vi "Circumference of Circle.vi"() -> ()   [LabVIEW 2020]
panel:
  out "Circumference":dbl
  in  "Radius":dbl
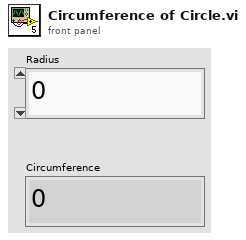
[diagram p1: front panel]
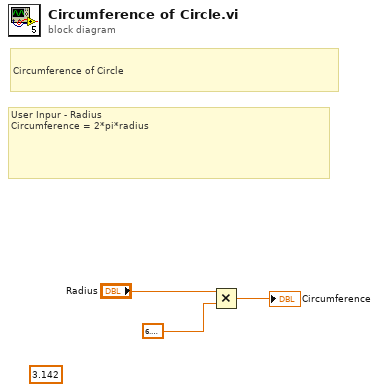
[diagram p0: block diagram]
diagram:
  (unwired) 3.142 ("y")
  # "User Inpur - Radius\nCircumference = 2*pi*radius"
  # "Circumference of Circle"
  n1 = Multiply(x="Radius", y=6.283185307179586) -> (x*y=→"Circumference":dbl)
